vi "Change Temperature_old.vi"(4 "error in":errorcluster, 6 "Rat(dlogR/dlogT)":dbl=0.66 format="%.2f", 7 "TempControl":bool[](array[boolean]), 8 "Current Field":dbl=9.0 format="%.2f", 9 "Temp Tolerance":dbl format="%.2f", 10 "Desired Temperature":dbl=305.0 format="%.2f", 11 "GPIB Address":u16=15 min=2 max=31 step=1) -> (0 "error out":errorcluster, 3 "Final Temp":dbl format="%.2f")   [LabVIEW 2020]
uses:
  Globals and TypeDefs/Type Definitions.llb/3 way Status.ctl
  Globals and TypeDefs/gStatus.vi
  Globals and TypeDefs/gTemperature.vi
panel:
  # "Temperature Controller Controls"
  # "Exist?"
  # "TC Enable or Monitor"
  # "Magneto-Correction?"
  # "Auto-Advancing?"
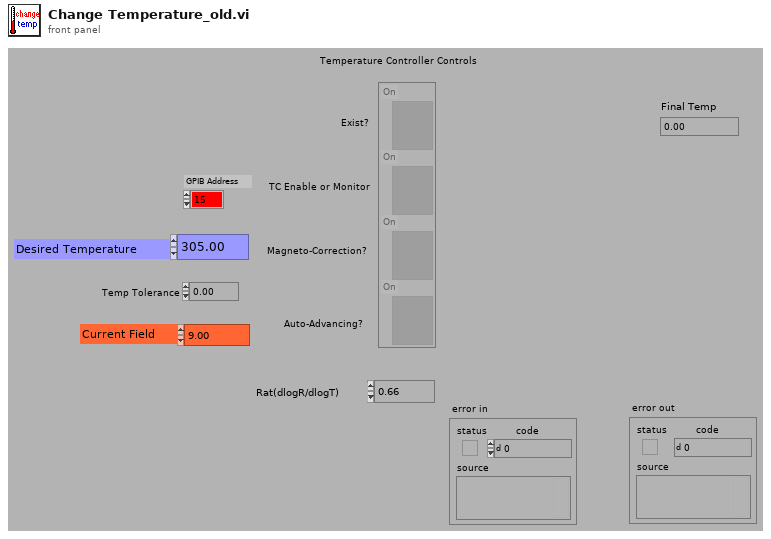
[diagram p1: front panel]
types:
  T1 = typedef "3 way Status.ctl" = u8
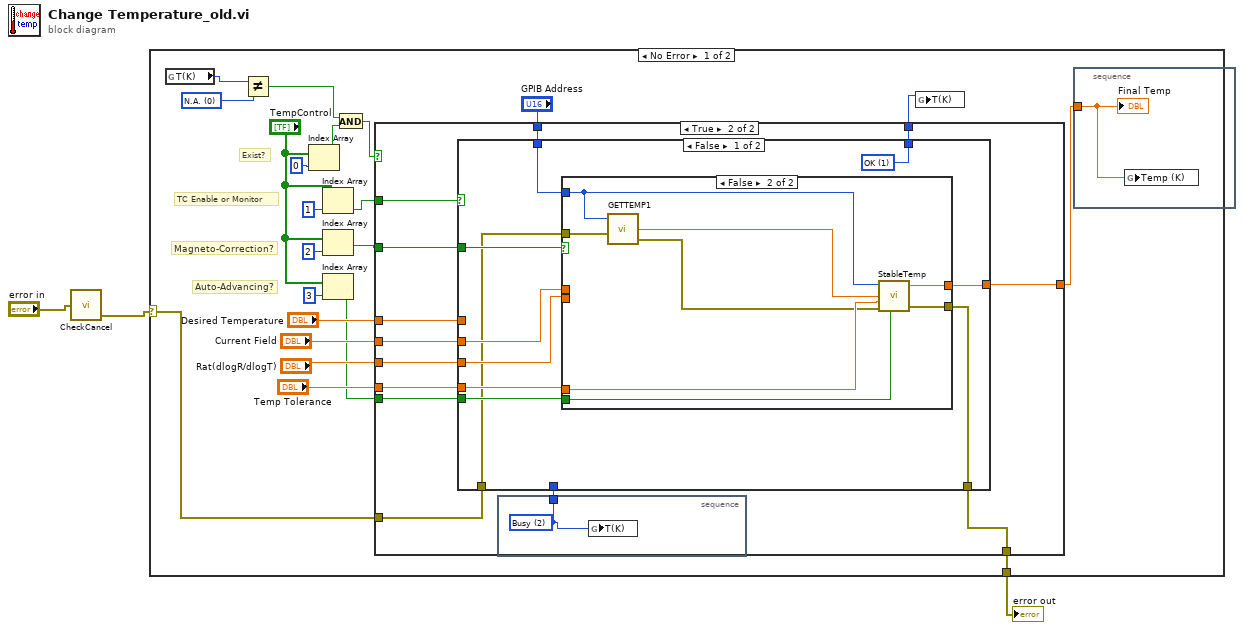
[diagram p0: block diagram]
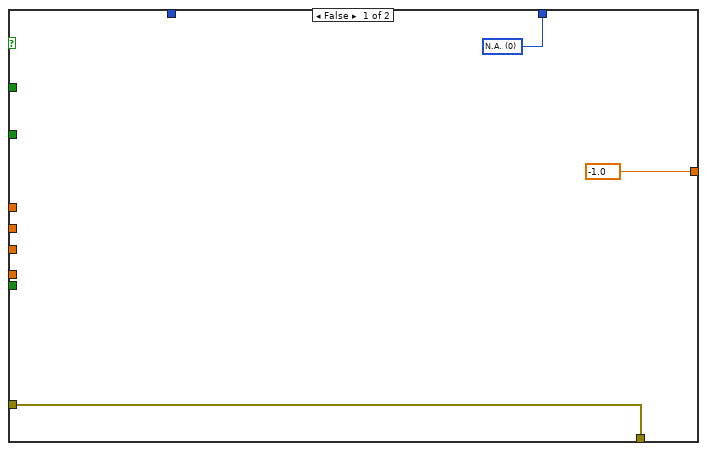
[diagram p2: hidden frame]
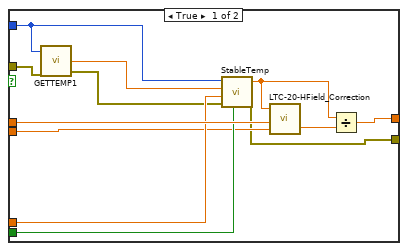
[diagram p3: hidden frame]
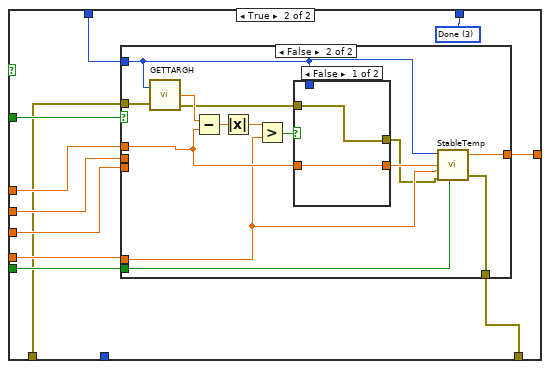
[diagram p4: hidden frame]
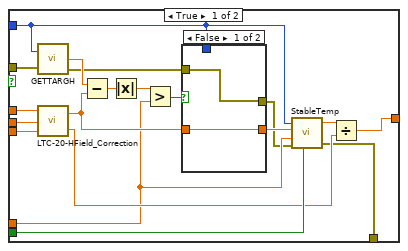
[diagram p5: hidden frame]
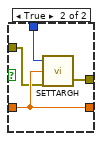
[diagram p6: hidden frame]
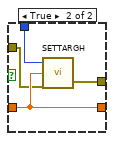
[diagram p7: hidden frame]
diagram:
  n1 = call "CheckCancel.vi"("error in (no error)"="error in") -> ("error out"=w3:errorcluster)  [unwired: 1 in, 1 out]
  n2 = case shown="No Error" w3 {
    selector: w3 -> [w5 w130]
    tunnel: [w4 w130] -> w1
    frame No Error {
      w11 = T1 0 items=["N.A.", "OK", "Busy", "Done"] ("y")
      # "Exist?"
      # "Auto-Advancing?"
      # "Magneto-Correction?"
      # "TC Enable or Monitor"
      n3 = global read "gStatus.vi" "T(K)"() -> (w7:T1)
      n4 = Not Equal?(x=w7, y=w11) -> (x != y?=w8:bool)
      n5 = Index Array(array="TempControl", index=0) -> (element=w10:bool)
      n6 = Index Array(array="TempControl", index=1) -> (element=w20:bool)
      n7 = Index Array(array="TempControl", index=2) -> (element=w15:bool)
      n8 = Index Array(array="TempControl", index=3) -> (element=w13:bool)
      n9 = And(x=w8, y=w10) -> (x .and. y?=w9:bool)
      n10 = case shown="True" w9 {
        tunnel: w20 -> [_ w42]
        tunnel: "Desired Temperature" -> [_ w41]
        tunnel: "Current Field" -> [_ w40]
        tunnel: "Rat(dlogR/dlogT)" -> [_ w39]
        tunnel: "GPIB Address" -> [_ w38]
        tunnel: w15 -> [_ w37]
        tunnel: "Temp Tolerance" -> [_ w36]
        tunnel: w13 -> [_ w35]
        tunnel: [-1.0 ("Final Temp") w34] -> w12
        tunnel: [w28 w33] -> w6
        tunnel: w5 -> [w27 w31]
        tunnel: [w27 w30] -> w4
        frame False {
          w28 = T1 0 items=["N.A.", "OK", "Busy", "Done"] ("y")
        }
        frame True {
          n11 = stacked-sequence {
            tunnel: [w43] -> w32
            frame #0 {
              w43 = T1 2 items=["N.A.", "OK", "Busy", "Done"] ("T(K)")
              n12 = global write "gStatus.vi" "T(K)"(w43) -> ()
            }
          }
          n13 = case shown="False" w42 {
            tunnel: w41 -> [_ w84]
            tunnel: w40 -> [w51 w83]
            tunnel: w39 -> [w50 w82]
            tunnel: w38 -> [w52 w81]
            tunnel: w37 -> [w53 w80]
            tunnel: w36 -> [w48 w79]
            tunnel: w35 -> [w49 w78]
            tunnel: [w47 w77] -> w34
            tunnel: w31 -> [w46 w76]
            tunnel: [w45 w75] -> w30
            tunnel: [w44 w74] -> w33
            tunnel: w32 -> [_ _]
            frame False {
              w44 = T1 1 items=["N.A.", "OK", "Busy", "Done"] ("T(K)")
              n14 = case shown="False" w53 {
                tunnel: w51 -> [w65 _]
                tunnel: w50 -> [w59 _]
                tunnel: w52 -> [w60 w70]
                tunnel: w48 -> [w64 w71]
                tunnel: w49 -> [w63 w73]
                tunnel: [w61 w72] -> w47
                tunnel: w46 -> [w56 w68]
                tunnel: [w54 w66] -> w45
                frame True {
                  n15 = call "GETTEMP1.VI"("GPIB Device"=w60, "error in (no error)"=w56) -> ("Sensor 1"=w58:sgl, "error out"=w55:errorcluster)  [unwired: 1 out]
                  n16 = call "StableTemp.VI"("GPIB Device"=w60, "Desired Temp"=w58, "Tolerance"=w64, "error in (no error)"=w55, "AutoAdvancing"=w63) -> ("Final Temp"=w57:sgl, "error out"=w54:errorcluster)  [unwired: 1 in]
                  n17 = call "LTC-20-HField_Correction.vi"("Rat(dlogR/dlogT)"=w59, "Current Field"=w65, "Desired Temperature"=w57) -> ("Correction Coef."=w62:dbl)  [unwired: 1 out]
                  n18 = Divide(x=w57, y=w62) -> (x/y=w61:dbl)
                }
                frame False {
                  n19 = call "GETTEMP1.VI"("GPIB Device"=w70, "error in (no error)"=w68) -> ("Sensor 1"=w69:sgl, "error out"=w67:errorcluster)  [unwired: 1 out]
                  n20 = call "StableTemp.VI"("GPIB Device"=w70, "Desired Temp"=w69, "Tolerance"=w71, "error in (no error)"=w67, "AutoAdvancing"=w73) -> ("Final Temp"=w72:sgl, "error out"=w66:errorcluster)  [unwired: 1 in]
                }
              }
            }
            frame True {
              w74 = T1 3 items=["N.A.", "OK", "Busy", "Done"] ("T(K)")
              n21 = case shown="False" w80 {
                tunnel: w84 -> [w103 w120]
                tunnel: w83 -> [w102 _]
                tunnel: w82 -> [w101 _]
                tunnel: w81 -> [w94 w118]
                tunnel: w79 -> [w87 w115]
                tunnel: w78 -> [w93 w117]
                tunnel: [w90 w114] -> w77
                tunnel: w76 -> [w89 w113]
                tunnel: [w85 w110] -> w75
                frame True {
                  n22 = call "GETTARGH.vi"("GPIB Device"=w94, "error in (no error)"=w89) -> ("Heater Setpoint"=w96:sgl, "error out"=w88:errorcluster)  [unwired: 1 out]
                  n23 = call "LTC-20-HField_Correction.vi"("Rat(dlogR/dlogT)"=w101, "Current Field"=w102, "Desired Temperature"=w103) -> ("Correction Coef."=w91:dbl, "TempSetpoint"=w97:dbl)
                  n24 = Subtract(x=w96, y=w97) -> (x-y=w100:dbl)
                  n25 = Absolute Value(x=w100) -> (abs(x)=w99:dbl)
                  n26 = Greater?(x=w99, y=w87) -> (0:w98:bool)
                  n27 = case shown="False" w98 {
                    tunnel: w97 -> [w105 w108]
                    tunnel: w94 -> [_ w109]
                    tunnel: [w105 w108] -> w95
                    tunnel: w88 -> [w104 w107]
                    tunnel: [w104 w106] -> w86
                    frame False {
                    }
                    frame True {
                      n28 = call "SETTARGH.vi"("error in (no error)"=w107, "Heater Setpoint"=w108, "GPIB Device"=w109) -> ("error out"=w106:errorcluster)  [unwired: 1 out]
                    }
                  }
                  n29 = call "StableTemp.VI"("GPIB Device"=w94, "Desired Temp"=w95, "Tolerance"=w87, "error in (no error)"=w86, "AutoAdvancing"=w93) -> ("Final Temp"=w92:sgl, "error out"=w85:errorcluster)  [unwired: 1 in]
                  n30 = Divide(x=w92, y=w91) -> (x/y=w90:dbl)
                }
                frame False {
                  n31 = call "GETTARGH.vi"("GPIB Device"=w118, "error in (no error)"=w113) -> ("Heater Setpoint"=w119:sgl, "error out"=w112:errorcluster)  [unwired: 1 out]
                  n32 = Subtract(x=w119, y=w120) -> (x-y=w123:dbl)
                  n33 = Absolute Value(x=w123) -> (abs(x)=w122:dbl)
                  n34 = Greater?(x=w122, y=w115) -> (0:w121:bool)
                  n35 = case shown="False" w121 {
                    tunnel: w120 -> [w125 w128]
                    tunnel: w118 -> [_ w129]
                    tunnel: [w125 w128] -> w116
                    tunnel: w112 -> [w124 w127]
                    tunnel: [w124 w126] -> w111
                    frame False {
                    }
                    frame True {
                      n36 = call "SETTARGH.vi"("error in (no error)"=w127, "Heater Setpoint"=w128, "GPIB Device"=w129) -> ("error out"=w126:errorcluster)  [unwired: 1 out]
                    }
                  }
                  n37 = call "StableTemp.VI"("GPIB Device"=w118, "Desired Temp"=w116, "Tolerance"=w115, "error in (no error)"=w111, "AutoAdvancing"=w117) -> ("Final Temp"=w114:sgl, "error out"=w110:errorcluster)  [unwired: 1 in]
                }
              }
            }
          }
        }
      }
      n38 = global write "gStatus.vi" "T(K)"(w6) -> ()
      n39 = stacked-sequence {
        tunnel: w12 -> [w26]
        frame #0 {
          n40 = global write "gTemperature.vi" "Temp (K)"(w26) -> ()
          "Final Temp" <- w26
        }
      }
    }
    frame Error {
    }
  }
  "error out" <- w1
